vi "Document API.vi"() -> ()   [LabVIEW 2017]
uses:
  LabVIEW NPOI/NPOI Document API/Document Type.ctl
  C:/Users/Neo/Desktop/Dev_Tools_BR/LabVIEW_NPOI/src/lib/NPOI 2.1.1/NPOI.dll
  lib/NPOI 2.1.1/NPOI.dll
  LabVIEW NPOI/NPOI Document API/Get Document Path.vi
  LabVIEW NPOI/NPOI Document API/Get Document Type.vi
  LabVIEW NPOI/NPOI Document API/Excel - Get Workbook Reference.vi
  LabVIEW NPOI/NPOI Document API/Excel - Get Worksheet Reference.vi
  LabVIEW NPOI/NPOI Document API/Document API.lvclass
panel:
  out "SheetName":string
  out "Document:Path":path
  out "Excel.Reference":refnum<k24>
  out "Document Type 2":T1
  out "Document Path":path
  in  "Document Type":T1
  in  "File Path":path
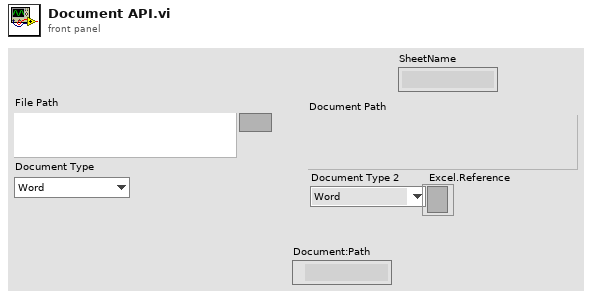
[diagram p1: front panel]
types:
  T1 = typedef "Document API.lvlib/Document API.lvclass/Document Type.ctl" = enum16{"Word", "Excel", "Undefined"}
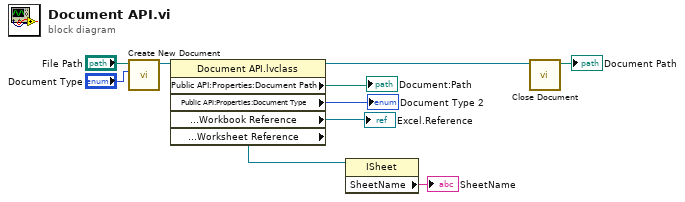
[diagram p0: block diagram]
diagram:
  n1 = call "Create New Document.vi"("Document Type"="Document Type", "File Path"="File Path") -> ("Document out"=w8:refnum<class "Document API.lvclass">)  [unwired: 8 in, 1 out]
  n2 = property class="Document API.lvclass"(reference=w8) -> (reference out=w6:refnum<class "Document API.lvclass">, "Public API:Properties:Document Path"=→"Document:Path":path, "Public API:Properties:Document Type"=→"Document Type 2":T1, "Public API:Properties:Excel.Workbook Reference"=→"Excel.Reference":refnum<k24>, "Public API:Properties:Excel.Worksheet Reference"=w3:refnum<k24>)  [unwired: 1 in, 1 out]
  n3 = property class="ISheet"(reference=w3) -> ("SheetName"=→"SheetName":string)  [unwired: 1 in, 2 out]
  n4 = call "Close Document.vi"("Document API in"=w6) -> ("Document Path"=→"Document Path":path)  [unwired: 9 in, 1 out]
